vi "Targets Mingle.vi"(1 "Single Targets":T5(array[cluster])) -> (0 "Married Targets":T4(array[cluster]))   [LabVIEW 2016]
panel:
  in  "Default target":T1
  in  "Cluster 2":T2
  in  "Particle Report":T3
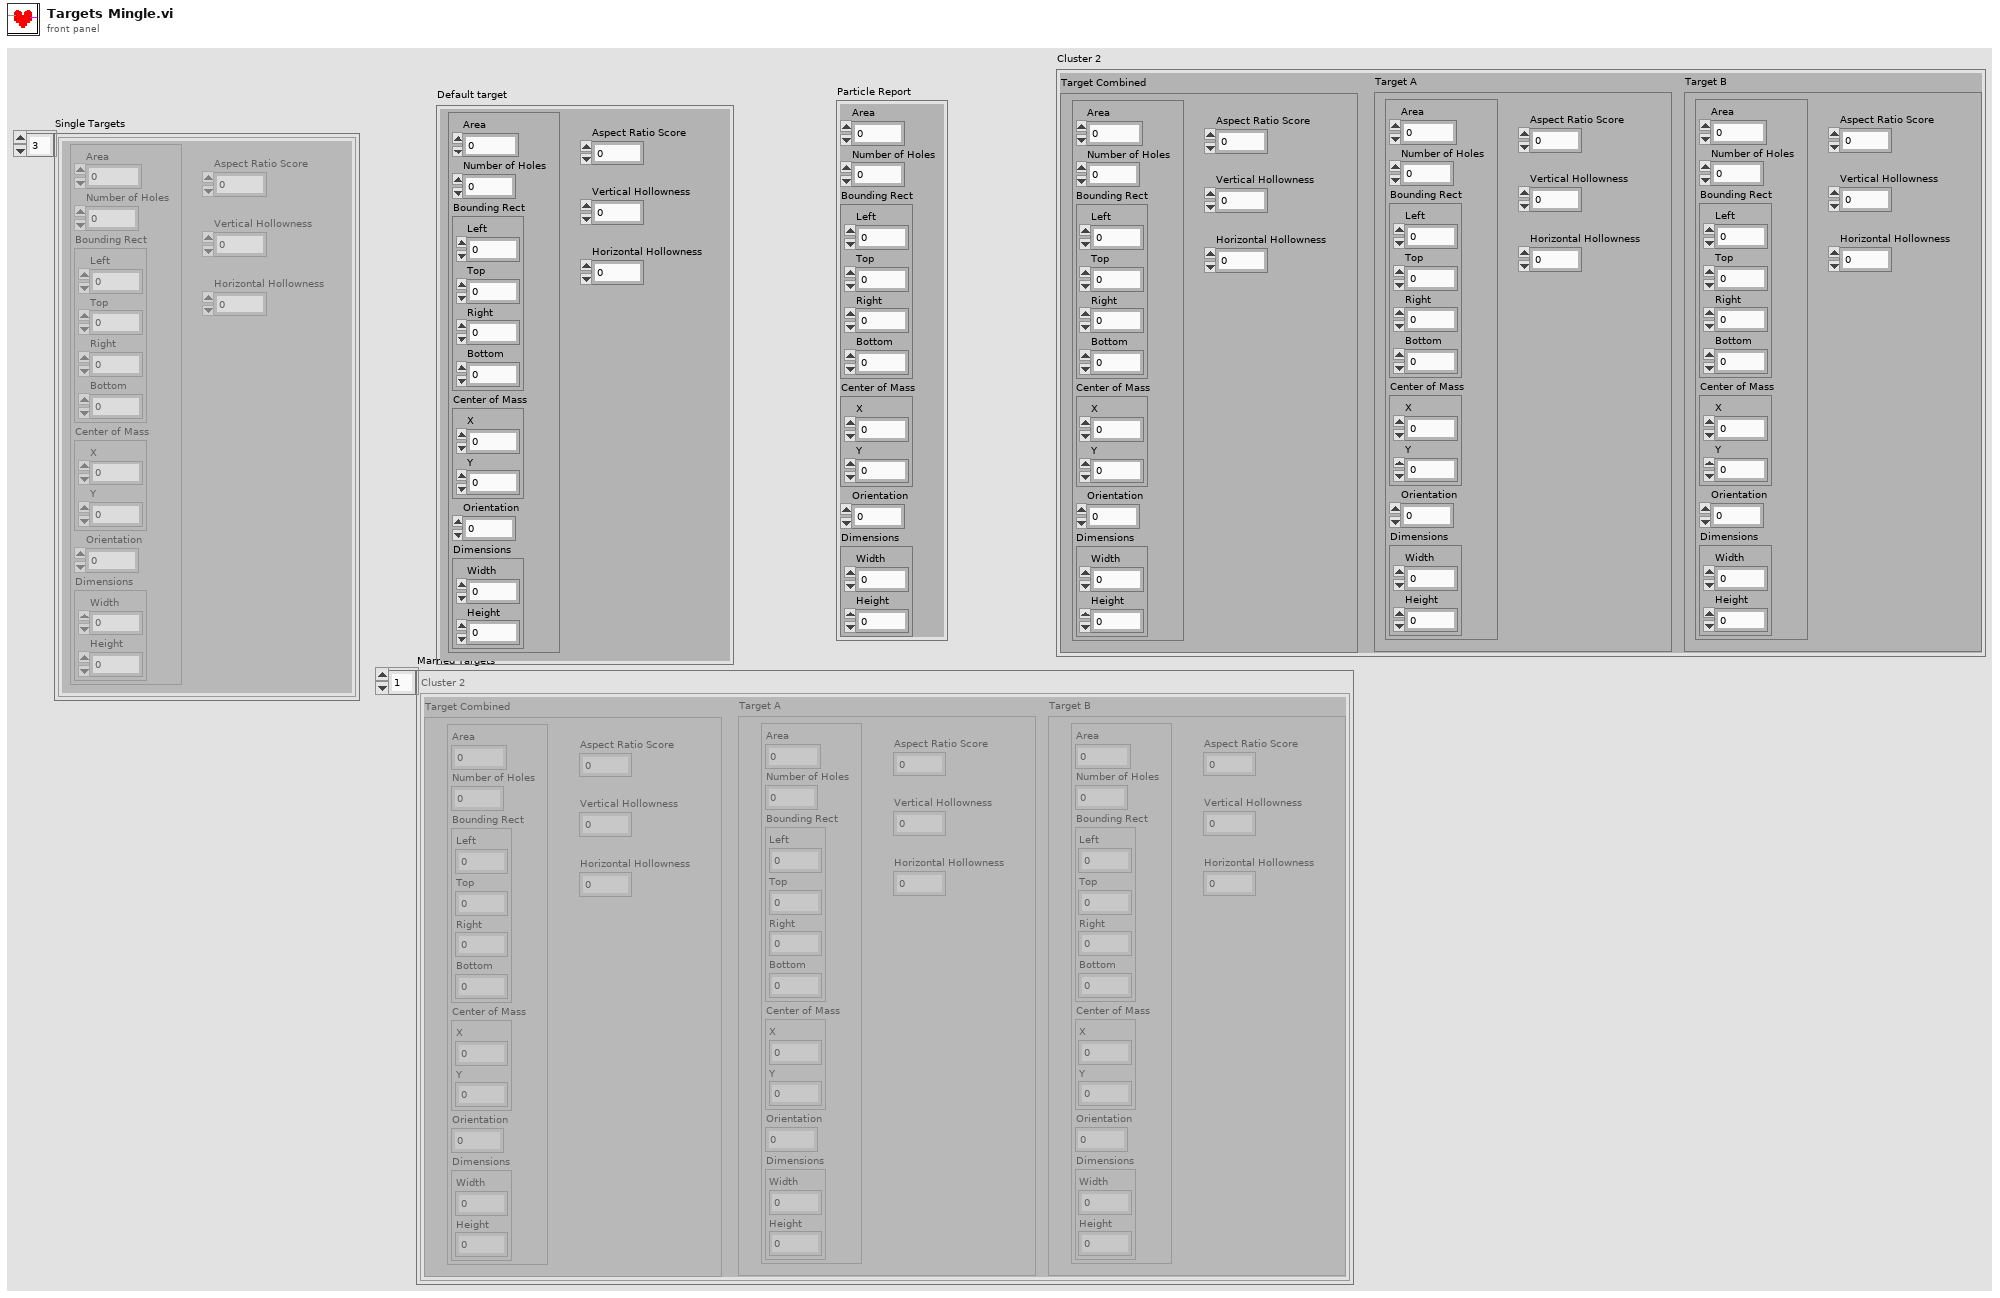
[diagram p1: front panel]
types:
  T1 = cluster{"Particle Report":cluster{"Area":dbl, "Number of Holes":dbl, "Bounding Rect":cluster{"Left":dbl, "Top":dbl, "Right":dbl, "Bottom":dbl}, "Center of Mass":cluster{"X":dbl, "Y":dbl}, "Orientation":dbl, "Dimensions":cluster{"Width":dbl, "Height":dbl}}, "Aspect Ratio Score":dbl, "Vertical Hollowness":dbl, "Horizontal Hollowness":dbl}
  T2 = cluster{"Target Combined":cluster{"Particle Report":cluster{"Area":dbl, "Number of Holes":dbl, "Bounding Rect":cluster{"Left":dbl, "Top":dbl, "Right":dbl, "Bottom":dbl}, "Center of Mass":cluster{"X":dbl, "Y":dbl}, "Orientation":dbl, "Dimensions":cluster{"Width":dbl, "Height":dbl}}, "Aspect Ratio Score":dbl, "Vertical Hollowness":dbl, "Horizontal Hollowness":dbl}, "Target A":cluster{"Particle Report":cluster{"Area":dbl, "Number of Holes":dbl, "Bounding Rect":cluster{"Left":dbl, "Top":dbl, "Right":dbl, "Bottom":dbl}, "Center of Mass":cluster{"X":dbl, "Y":dbl}, "Orientation":dbl, "Dimensions":cluster{"Width":dbl, "Height":dbl}}, "Aspect Ratio Score":dbl, "Vertical Hollowness":dbl, "Horizontal Hollowness":dbl}, "Target B":cluster{"Particle Report":cluster{"Area":dbl, "Number of Holes":dbl, "Bounding Rect":cluster{"Left":dbl, "Top":dbl, "Right":dbl, "Bottom":dbl}, "Center of Mass":cluster{"X":dbl, "Y":dbl}, "Orientation":dbl, "Dimensions":cluster{"Width":dbl, "Height":dbl}}, "Aspect Ratio Score":dbl, "Vertical Hollowness":dbl, "Horizontal Hollowness":dbl}}
  T3 = cluster{"Area":dbl, "Number of Holes":dbl, "Bounding Rect":cluster{"Left":dbl, "Top":dbl, "Right":dbl, "Bottom":dbl}, "Center of Mass":cluster{"X":dbl, "Y":dbl}, "Orientation":dbl, "Dimensions":cluster{"Width":dbl, "Height":dbl}}
  T4 = cluster{"Target Combined":cluster{"Particle Report":cluster{"Area":dbl, "Number of Holes":dbl, "Bounding Rect":cluster{"Left":dbl, "Top":dbl, "Right":dbl, "Bottom":dbl}, "Center of Mass":cluster{"X":dbl, "Y":dbl}, "Orientation":dbl, "Dimensions":cluster{"Width":dbl, "Height":dbl}}, "Aspect Ratio Score":dbl, "Vertical Hollowness":dbl, "Horizontal Hollowness":dbl}, "Target A":cluster{"Particle Report":cluster{"Area":dbl, "Number of Holes":dbl, "Bounding Rect":cluster{"Left":dbl, "Top":dbl, "Right":dbl, "Bottom":dbl}, "Center of Mass":cluster{"X":dbl, "Y":dbl}, "Orientation":dbl, "Dimensions":cluster{"Width":dbl, "Height":dbl}}, "Aspect Ratio Score":dbl, "Vertical Hollowness":dbl, "Horizontal Hollowness":dbl}, "Target B":cluster{"Particle Report":cluster{"Area":dbl, "Number of Holes":dbl, "Bounding Rect":cluster{"Left":dbl, "Top":dbl, "Right":dbl, "Bottom":dbl}, "Center of Mass":cluster{"X":dbl, "Y":dbl}, "Orientation":dbl, "Dimensions":cluster{"Width":dbl, "Height":dbl}}, "Aspect Ratio Score":dbl, "Vertical Hollowness":dbl, "Horizontal Hollowness":dbl}}[]
  T5 = cluster{"Particle Report":cluster{"Area":dbl, "Number of Holes":dbl, "Bounding Rect":cluster{"Left":dbl, "Top":dbl, "Right":dbl, "Bottom":dbl}, "Center of Mass":cluster{"X":dbl, "Y":dbl}, "Orientation":dbl, "Dimensions":cluster{"Width":dbl, "Height":dbl}}, "Aspect Ratio Score":dbl, "Vertical Hollowness":dbl, "Horizontal Hollowness":dbl}[]
  T6 = cluster{"Left":dbl, "Top":dbl, "Right":dbl, "Bottom":dbl}
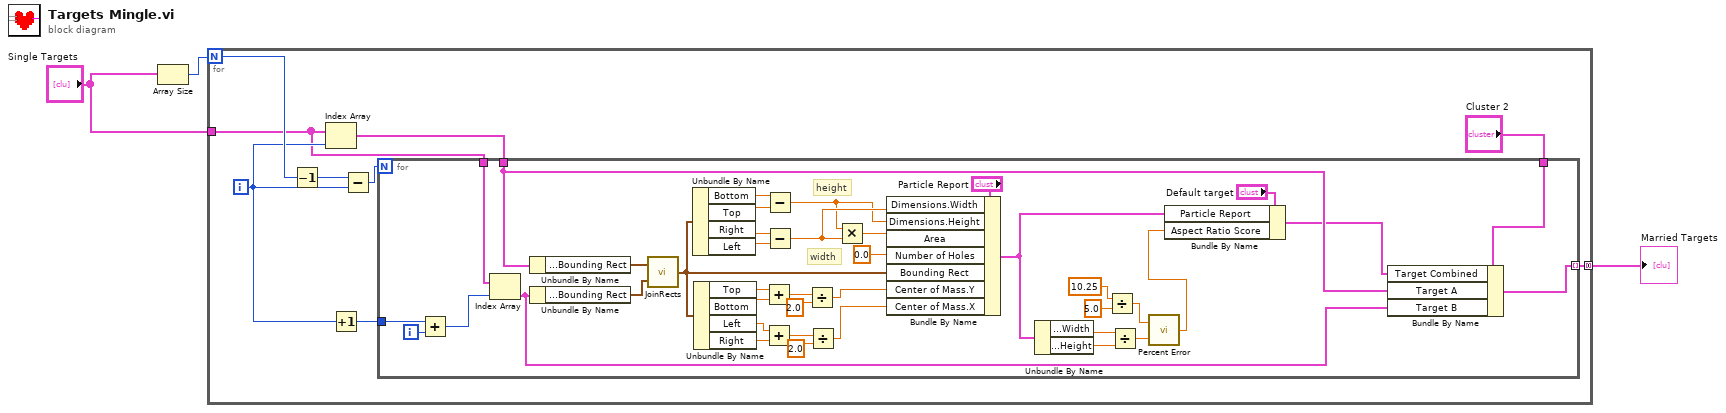
[diagram p0: block diagram]
diagram:
  n1 = Array Size(array="Single Targets") -> (size(s)=w3:i32)
  n2 = for {
    N: w3 -> [w11]
    tunnel: "Single Targets" -> [w4]
    tunnel: [w6] -> w1 mode=concatenating
    i -> [w10]
    n3 = Decrement(x=w11) -> (x-1=w12:i32)
    n4 = Index Array(array=w4, index=w10) -> (element=w8:T1)
    n5 = Increment(x=w10) -> (x+1=w9:i32)
    n6 = Subtract(x=w12, y=w10) -> (x-y=w5:i32)
    n7 = for {
      N: w5 -> [_]
      tunnel: w9 -> [w52]
      tunnel: w4 -> [w49]
      tunnel: w8 -> [w18]
      tunnel: "Cluster 2" -> [w48]
      tunnel: [w20] -> w6 mode=indexing
      i -> [w51]
      # "height"
      # "width"
      n8 = Add(x=w52, y=w51) -> (x+y=w50:i32)
      n9 = Index Array(array=w49, index=w50) -> (element=w17:T1)
      n10 = Unbundle By Name(w18) -> ("Particle Report.Bounding Rect"=w47:T6)
      n11 = Unbundle By Name(w17) -> ("Particle Report.Bounding Rect"=w46:T6)
      n12 = call "JoinRects.vi"("Rect in 2"=w46, "Rect in 1"=w47) -> ("Rect out"=w37:T6)
      n13 = Unbundle By Name(w37) -> ("Bottom"=w45:dbl, "Top"=w44:dbl, "Right"=w43:dbl, "Left"=w42:dbl)
      n14 = Unbundle By Name(w37) -> ("Top"=w36:dbl, "Bottom"=w35:dbl, "Left"=w30:dbl, "Right"=w29:dbl)
      n15 = Add(x=w36, y=w35) -> (x+y=w33:dbl)
      n16 = Add(x=w30, y=w29) -> (x+y=w31:dbl)
      n17 = Subtract(x=w45, y=w44) -> (x-y=w39:dbl)
      n18 = Subtract(x=w43, y=w42) -> (x-y=w40:dbl)
      n19 = Divide(x=w33, y=2.0) -> (x/y=w28:dbl)
      n20 = Divide(x=w31, y=2.0) -> (x/y=w27:dbl)
      n21 = Multiply(x=w39, y=w40) -> (x*y=w41:dbl)
      n22 = Bundle By Name(cluster="Particle Report", "Dimensions.Width"=w40, "Dimensions.Height"=w39, "Area"=w41, "Number of Holes"=0.0, "Bounding Rect"=w37, "Center of Mass.Y"=w28, "Center of Mass.X"=w27) -> (w15:T3)
      n23 = Unbundle By Name(w15) -> ("Dimensions.Width"=w22:dbl, "Dimensions.Height"=w21:dbl)
      n24 = Divide(x=10.25, y=5.0) -> (x/y=w25:dbl)
      n25 = Divide(x=w22, y=w21) -> (x/y=w26:dbl)
      n26 = call "Percent Error.vi"("Measured Values"=w26, "Accepted Value"=w25) -> ("Percent Error"=w14:dbl)
      n27 = Bundle By Name(cluster="Default target", "Particle Report"=w15, "Aspect Ratio Score"=w14) -> (w13:T1)
      n28 = Bundle By Name(cluster=w48, "Target Combined"=w13, "Target A"=w18, "Target B"=w17) -> (w20:T2)
    }
  }
  "Married Targets" <- w1
